vi "GSIOCimmediate.vi"(4 "Timeout (ms)":i32=2000, 5 "Max":i32=20, 6 "Command":string, 7 "ID":i32) -> (2 "Response":string, 3 "ID out":i32)   [LabVIEW 2012]
uses:
  Gsioc32.dll
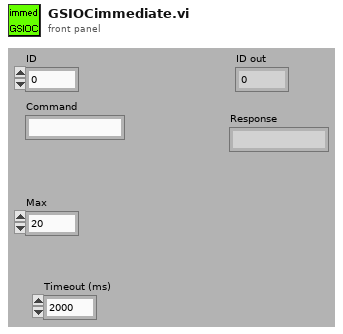
[diagram p1: front panel]
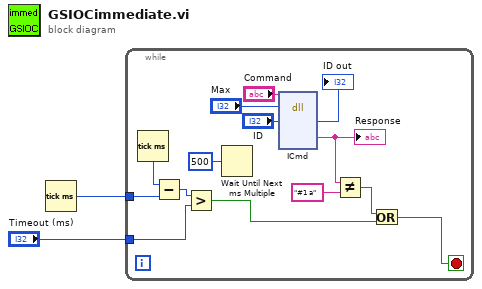
[diagram p0: block diagram]
diagram:
  n1 = Tick Count (ms)() -> (millisecond timer value=w2:u32)
  n2 = while {
    tunnel: w2 -> [w9]
    tunnel: "Timeout (ms)" -> [w7]
    stop <- w4 stop-if-true
    n3 = Tick Count (ms)() -> (millisecond timer value=w10:u32)
    n4 = Subtract(x=w10, y=w9) -> (x-y=w8:u32)
    n5 = Greater?(x=w8, y=w7) -> (0:w5:bool)
    n6 = Wait Until Next ms Multiple(millisecond multiple=u32 500) -> ()  [unwired: 1 out]
    n7 = dll-call lib="C:/WINDOWS/SYSTEM32/Gsioc32.dll" fn="ICmd"("ID"="ID", "Cmd"="Command", "Max"="Max") -> ("ID"=→"ID out":i32, "Rsp"=w12:string)  [unwired: 7 in, 2 out]
    "Response" <- w12
    n8 = Not Equal?(x=w12, y="#1 a") -> (x != y?=w6:bool)
    n9 = Or(x=w6, y=w5) -> (x .or. y?=w4:bool)
  }
